vi "First Word Statistics by Any.vi"(11 "Dictionary":string[](array[string])) -> (3 "Word Statistic":T1[](array[typedef]))   [LabVIEW 2015]
uses:
  TypeDef/Word Statistic.ctl
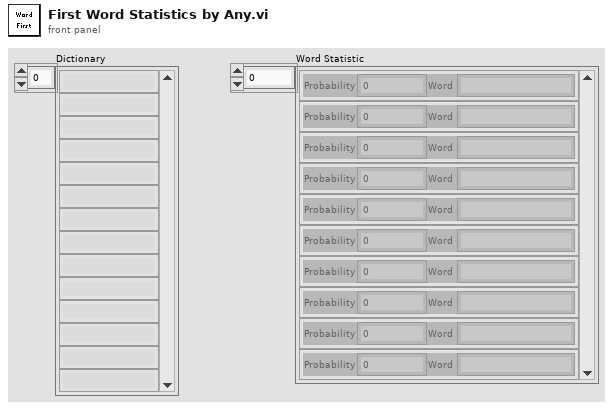
[diagram p1: front panel]
types:
  T1 = typedef "Word Statistic.ctl" = cluster{"Probability":dbl, "Word":string}
  T2 = typedef "Letter Statistic.ctl" = cluster{"Letter":string, "any":dbl, "1":dbl, "2":dbl, "3":dbl, "4":dbl, "5":dbl}
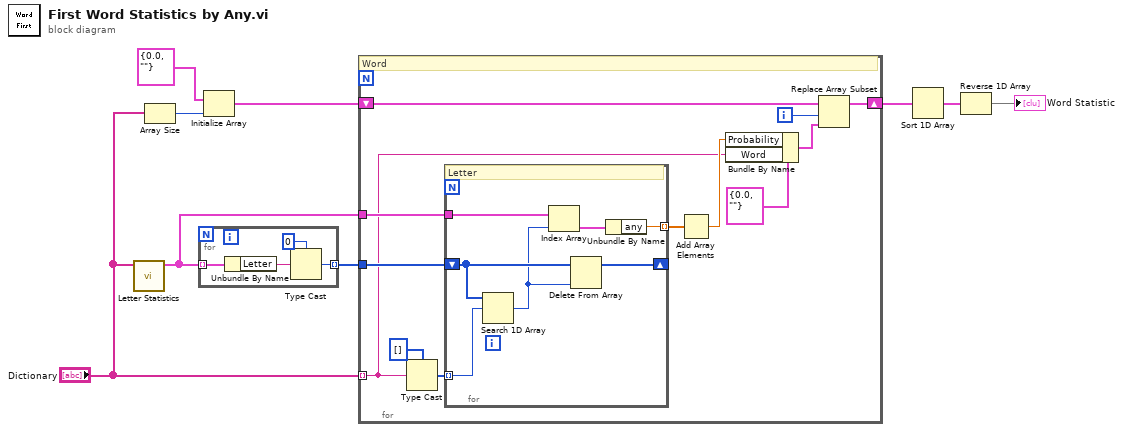
[diagram p0: block diagram]
diagram:
  n1 = call "Letter Statistics.vi"("Dictionary"="Dictionary") -> ("Statistic"=w8:T2[])  [unwired: 10 in]
  n2 = Array Size(array="Dictionary") -> (size(s)=w6:i32)
  n3 = for {
    tunnel: w8 -> [w13] mode=indexing
    tunnel: [w11] -> w9 mode=indexing
    n4 = Unbundle By Name(w13) -> ("Letter"=w10:string)
    n5 = Type Cast(type=u8 0, x=w10) -> (*(type *) &x=w11:u8)
  }
  n6 = Initialize Array(T1 {"Probability"=0.0, "Word"=""} ("Word Statistic"), w6) -> (w4:T1[])
  n7 = for {
    tunnel: "Dictionary" -> [w14] mode=indexing
    tunnel: w8 -> [w25]
    tunnel: w9 -> [w24]
    shift-right: [w19] -> w2
    shift-left: w4 -> [w20]
    i -> [w17]
    # "Word"
    n8 = Type Cast(type=u8[] [] ("letter"), x=w14) -> (*(type *) &x=w23:u8[])
    n9 = for {
      tunnel: w23 -> [w32] mode=indexing
      tunnel: w25 -> [w31]
      tunnel: [w29] -> w16 mode=indexing
      shift-right: [w27] -> _
      shift-left: w24 -> [w28]
      # "Letter"
      n10 = Search 1D Array(1D array=w28, element=w32) -> (index of element=w26:i32)  [unwired: 1 in]
      n11 = Index Array(array=w31, index=w26) -> (element=w30:T2)
      n12 = Delete From Array(array=w28, index=w26) -> (array with subset deleted=w27:u8[])  [unwired: 1 in, 1 out]
      n13 = Unbundle By Name(w30) -> ("any"=w29:dbl)
    }
    n14 = Add Array Elements(numeric array=w16) -> (sum=w15:dbl)
    n15 = Bundle By Name(cluster=T1 {"Probability"=0.0, "Word"=""} ("Word Statistic"), "Probability"=w15, "Word"=w14) -> (w18:T1)
    n16 = Replace Array Subset(array=w20, new element=w18, index=w17) -> (w19:T1[])
  }
  n17 = Sort 1D Array(array=w2) -> (sorted array=w3:T1[])
  n18 = Reverse 1D Array(array=w3) -> (reversed array=→"Word Statistic":T1[])
